vi "DriverStationSendData.vi"   [LabVIEW 2020]
doc: "This VI continously sends data from the robot to the FRC 4265 Dashboard, the joysticks, and the FIRST Driver Station. Data are only sent to the network tables when values change. Detailed sensor data are only sent when the user is currently viewing the Tune tab on the FRC 4265 Dashboard."
uses:
  586985d1-6105-46df-bd9b-6f07d21ed352.vi
  9d68b025-fd20-40c1-968a-0b15d20a54dd.vi
  423974b0-4a7b-493f-bebd-78b7d8b4919e.vi
  195aadaf-e727-4ba4-8a8c-fe9315911b93.vi
  fd66a432-e6c7-4ce8-9440-e2a32478c4e6.vi
  a01e8785-2e45-445a-ba95-97aad2eef7fd.vi
  f8967374-96a0-4ff7-9b39-d84b703c09a6.vi
  36759aca-d9c6-44a3-918a-9a0e895c718f.vi
  d2dc3f3f-39b5-4c17-a933-05bbedc8d5d9.vi
  47e8091e-0604-4560-b6ee-932fcc40f94c.vi
  040c557e-2b24-4d13-8fef-d98c711cf45f.vi
  6883bb39-9618-44d1-87fc-0a8820399f5c.vi
  c8eef334-f098-4cd9-9ea5-5d5092550f38.vi
  89115614-314f-44eb-b4c5-fafba5d31cd4.vi
  7dbbd9ae-9e42-48a3-962d-7503ed9ff88f.vi
  f31b310c-46e7-4cd5-9fe8-a6567badd324.vi
  9f98788f-6f1b-4a83-a100-7d872b9f460c.vi
  d5b4d43d-cd94-4278-ad04-5030dc28ac17.vi
  90b8ffb3-02b0-4f37-8578-c415475fcf1f.vi
  26471c2c-aca7-4047-a7cd-e40da11d04c1.vi
  839d0640-05f3-423d-909c-b7036ab13647.vi
  04c53935-f0da-44ec-a78a-2e7adf0baac3.vi
  e4b3569e-220c-43b1-9843-603dbcb8d192.vi
  0c9c2ce5-4f8f-4d2f-a61f-dde9fdddd21a.vi
  948ebb5e-1fee-45f5-b788-843df8d92f11.vi
  07cec073-88f4-4f05-94a3-d05e12405c4e.vi
  c10cd8a7-bdb7-4c92-ac5c-00af4ab7dc85.vi
  ce82ba1c-dcc2-498f-8d23-146b12230de2.vi
  6245c486-c412-4e37-a41a-fc8346b5d865.vi
  15bc976b-cae7-4018-a285-3ceb7c36b13a.vi
  cbbdf295-aa1d-4db8-8566-cac5820e4458.vi
  52d993e2-6fbc-4ee4-b085-b3f80a4c3067.vi
  5ccc8aa6-325d-4660-b060-52e30b1d582a.vi
  296afef1-bc02-48ee-92b6-09523bb21575.vi
  811948b9-57e2-4f47-a6f6-f2932d14082f.vi
  5739ca73-a30d-4c92-9c50-72d6edc45fc4.vi
  0620df73-5841-450f-a219-dd10bb38cbc0.vi
  fb087c59-fbb1-4979-ba7d-d29f083bcd8a.vi
  94826c24-d30e-4eee-b4d4-6d626a9b9fe7.vi
  fa7611ee-6daf-4341-84ec-bae2216748b8.vi
  db54ab23-5628-4d32-8d99-5ed0975ac3fe.vi
  8f6ab1f9-5983-4917-be41-7b146f8af2a0.vi
  4287b2c4-d12d-433b-80b7-0e569e2acc2b.vi
  011bd4f8-b5d7-4f12-8be3-d50395e1dcf1.vi
  f674d2d5-6a94-4f89-a0c2-325738beccea.vi
  281bad53-2b02-4799-afd8-5b44cc752506.vi
  47b7797c-6abd-448a-a8c1-ba6fc8ec09e7.vi
  65b8bab8-f184-4713-b917-96f68816fcd7.vi
  e783cd06-363b-4b9f-976c-53354950d7da.vi
  6a204843-18fb-45b9-b066-5e86b1c86445.vi
  0f67704b-983f-40f8-b984-26854eaa7ede.vi
  72a9b6b9-5c07-430f-a317-8ae0f710e1b8.vi
  d6d4123b-2723-46fe-ae0c-2abe92ccdc7f.vi
  7889d354-fa55-478c-b42d-730a5990e710.vi
  09f305fd-a7e8-43a8-8a10-94883e021016.vi
  f11304fe-b25d-4509-a679-e814399fdb49.vi
  d69f5ca2-9cc8-4f10-9e43-09bf58b41655.vi
  fa6aa2a5-b57b-4d46-802a-52895c79f189.vi
  1761f515-972c-49cd-8d46-35dcec4c579e.vi
  14433321-cc0b-4c86-996a-891af0111116.vi
  665401e1-7162-4411-af45-b6d951c7e0b0.vi
  7b6a1411-5027-49fa-871d-ec9f81e31f95.vi
  20dd8ad3-6bbc-4cac-b559-7f798e2b6680.vi
  5e95d400-1295-40c5-af46-ec5444c3a2ff.vi
  d5b53c9f-0752-48c4-83e9-94c6e20357af.vi
  a2a431f6-075f-4920-bddd-4a0a2690fbc3.vi
  755407eb-a184-43a3-8213-370691478bd6.vi
  293bca24-914b-4f92-b125-1f9f12182447.vi
  63edfc8b-2713-4fb9-bbf0-712b13f7ed91.vi
  5dc304d7-e71b-4cd2-8d9d-954937278b50.vi
  c0b3d222-824d-4eea-b194-4551ccfede72.vi
  c227876e-c49d-4561-a8c1-0ac62d9f5df0.vi
  e617f737-58a4-4889-9924-01a8da667f92.vi
  e9fd310d-87c6-4082-92c8-bcf79789ccf6.vi
  f0969710-38cf-416a-9d18-6a527ee639e4.vi
  a9076398-35a2-42a7-b542-3dd64d126b59.vi
  44842b00-b9c8-4b1f-a6e0-fc22f00ef89a.vi
  586985d1-6105-46df-bd9b-6f07d21ed352.vi/77c742ae-e671-49bb-a825-a6e8cebc9f63.vi
  9d68b025-fd20-40c1-968a-0b15d20a54dd.vi/77c742ae-e671-49bb-a825-a6e8cebc9f63.vi
  423974b0-4a7b-493f-bebd-78b7d8b4919e.vi/77c742ae-e671-49bb-a825-a6e8cebc9f63.vi
  195aadaf-e727-4ba4-8a8c-fe9315911b93.vi/77c742ae-e671-49bb-a825-a6e8cebc9f63.vi
  fd66a432-e6c7-4ce8-9440-e2a32478c4e6.vi/77c742ae-e671-49bb-a825-a6e8cebc9f63.vi
  a01e8785-2e45-445a-ba95-97aad2eef7fd.vi/77c742ae-e671-49bb-a825-a6e8cebc9f63.vi
  f8967374-96a0-4ff7-9b39-d84b703c09a6.vi/77c742ae-e671-49bb-a825-a6e8cebc9f63.vi
  36759aca-d9c6-44a3-918a-9a0e895c718f.vi/77c742ae-e671-49bb-a825-a6e8cebc9f63.vi
  d2dc3f3f-39b5-4c17-a933-05bbedc8d5d9.vi/77c742ae-e671-49bb-a825-a6e8cebc9f63.vi
  47e8091e-0604-4560-b6ee-932fcc40f94c.vi/77c742ae-e671-49bb-a825-a6e8cebc9f63.vi
  040c557e-2b24-4d13-8fef-d98c711cf45f.vi/77c742ae-e671-49bb-a825-a6e8cebc9f63.vi
  6883bb39-9618-44d1-87fc-0a8820399f5c.vi/77c742ae-e671-49bb-a825-a6e8cebc9f63.vi
  c8eef334-f098-4cd9-9ea5-5d5092550f38.vi/77c742ae-e671-49bb-a825-a6e8cebc9f63.vi
  89115614-314f-44eb-b4c5-fafba5d31cd4.vi/77c742ae-e671-49bb-a825-a6e8cebc9f63.vi
  7dbbd9ae-9e42-48a3-962d-7503ed9ff88f.vi/77c742ae-e671-49bb-a825-a6e8cebc9f63.vi
  f31b310c-46e7-4cd5-9fe8-a6567badd324.vi/77c742ae-e671-49bb-a825-a6e8cebc9f63.vi
  9f98788f-6f1b-4a83-a100-7d872b9f460c.vi/77c742ae-e671-49bb-a825-a6e8cebc9f63.vi
  d5b4d43d-cd94-4278-ad04-5030dc28ac17.vi/77c742ae-e671-49bb-a825-a6e8cebc9f63.vi
  90b8ffb3-02b0-4f37-8578-c415475fcf1f.vi/77c742ae-e671-49bb-a825-a6e8cebc9f63.vi
  26471c2c-aca7-4047-a7cd-e40da11d04c1.vi/77c742ae-e671-49bb-a825-a6e8cebc9f63.vi
  839d0640-05f3-423d-909c-b7036ab13647.vi/77c742ae-e671-49bb-a825-a6e8cebc9f63.vi
  04c53935-f0da-44ec-a78a-2e7adf0baac3.vi/77c742ae-e671-49bb-a825-a6e8cebc9f63.vi
  e4b3569e-220c-43b1-9843-603dbcb8d192.vi/77c742ae-e671-49bb-a825-a6e8cebc9f63.vi
  0c9c2ce5-4f8f-4d2f-a61f-dde9fdddd21a.vi/77c742ae-e671-49bb-a825-a6e8cebc9f63.vi
  948ebb5e-1fee-45f5-b788-843df8d92f11.vi/77c742ae-e671-49bb-a825-a6e8cebc9f63.vi
  07cec073-88f4-4f05-94a3-d05e12405c4e.vi/77c742ae-e671-49bb-a825-a6e8cebc9f63.vi
  c10cd8a7-bdb7-4c92-ac5c-00af4ab7dc85.vi/77c742ae-e671-49bb-a825-a6e8cebc9f63.vi
  ce82ba1c-dcc2-498f-8d23-146b12230de2.vi/77c742ae-e671-49bb-a825-a6e8cebc9f63.vi
  6245c486-c412-4e37-a41a-fc8346b5d865.vi/77c742ae-e671-49bb-a825-a6e8cebc9f63.vi
  15bc976b-cae7-4018-a285-3ceb7c36b13a.vi/77c742ae-e671-49bb-a825-a6e8cebc9f63.vi
  cbbdf295-aa1d-4db8-8566-cac5820e4458.vi/77c742ae-e671-49bb-a825-a6e8cebc9f63.vi
  52d993e2-6fbc-4ee4-b085-b3f80a4c3067.vi/77c742ae-e671-49bb-a825-a6e8cebc9f63.vi
  5ccc8aa6-325d-4660-b060-52e30b1d582a.vi/77c742ae-e671-49bb-a825-a6e8cebc9f63.vi
  296afef1-bc02-48ee-92b6-09523bb21575.vi/77c742ae-e671-49bb-a825-a6e8cebc9f63.vi
  811948b9-57e2-4f47-a6f6-f2932d14082f.vi/77c742ae-e671-49bb-a825-a6e8cebc9f63.vi
  5739ca73-a30d-4c92-9c50-72d6edc45fc4.vi/77c742ae-e671-49bb-a825-a6e8cebc9f63.vi
  0620df73-5841-450f-a219-dd10bb38cbc0.vi/77c742ae-e671-49bb-a825-a6e8cebc9f63.vi
  fb087c59-fbb1-4979-ba7d-d29f083bcd8a.vi/77c742ae-e671-49bb-a825-a6e8cebc9f63.vi
  94826c24-d30e-4eee-b4d4-6d626a9b9fe7.vi/77c742ae-e671-49bb-a825-a6e8cebc9f63.vi
  fa7611ee-6daf-4341-84ec-bae2216748b8.vi/77c742ae-e671-49bb-a825-a6e8cebc9f63.vi
  db54ab23-5628-4d32-8d99-5ed0975ac3fe.vi/77c742ae-e671-49bb-a825-a6e8cebc9f63.vi
  8f6ab1f9-5983-4917-be41-7b146f8af2a0.vi/77c742ae-e671-49bb-a825-a6e8cebc9f63.vi
  4287b2c4-d12d-433b-80b7-0e569e2acc2b.vi/77c742ae-e671-49bb-a825-a6e8cebc9f63.vi
  011bd4f8-b5d7-4f12-8be3-d50395e1dcf1.vi/77c742ae-e671-49bb-a825-a6e8cebc9f63.vi
  f674d2d5-6a94-4f89-a0c2-325738beccea.vi/77c742ae-e671-49bb-a825-a6e8cebc9f63.vi
  281bad53-2b02-4799-afd8-5b44cc752506.vi/77c742ae-e671-49bb-a825-a6e8cebc9f63.vi
  47b7797c-6abd-448a-a8c1-ba6fc8ec09e7.vi/77c742ae-e671-49bb-a825-a6e8cebc9f63.vi
  65b8bab8-f184-4713-b917-96f68816fcd7.vi/77c742ae-e671-49bb-a825-a6e8cebc9f63.vi
  e783cd06-363b-4b9f-976c-53354950d7da.vi/77c742ae-e671-49bb-a825-a6e8cebc9f63.vi
  6a204843-18fb-45b9-b066-5e86b1c86445.vi/77c742ae-e671-49bb-a825-a6e8cebc9f63.vi
  0f67704b-983f-40f8-b984-26854eaa7ede.vi/77c742ae-e671-49bb-a825-a6e8cebc9f63.vi
  72a9b6b9-5c07-430f-a317-8ae0f710e1b8.vi/77c742ae-e671-49bb-a825-a6e8cebc9f63.vi
  d6d4123b-2723-46fe-ae0c-2abe92ccdc7f.vi/77c742ae-e671-49bb-a825-a6e8cebc9f63.vi
  7889d354-fa55-478c-b42d-730a5990e710.vi/77c742ae-e671-49bb-a825-a6e8cebc9f63.vi
  09f305fd-a7e8-43a8-8a10-94883e021016.vi/77c742ae-e671-49bb-a825-a6e8cebc9f63.vi
  f11304fe-b25d-4509-a679-e814399fdb49.vi/77c742ae-e671-49bb-a825-a6e8cebc9f63.vi
  d69f5ca2-9cc8-4f10-9e43-09bf58b41655.vi/77c742ae-e671-49bb-a825-a6e8cebc9f63.vi
  fa6aa2a5-b57b-4d46-802a-52895c79f189.vi/77c742ae-e671-49bb-a825-a6e8cebc9f63.vi
  1761f515-972c-49cd-8d46-35dcec4c579e.vi/77c742ae-e671-49bb-a825-a6e8cebc9f63.vi
  14433321-cc0b-4c86-996a-891af0111116.vi/77c742ae-e671-49bb-a825-a6e8cebc9f63.vi
  665401e1-7162-4411-af45-b6d951c7e0b0.vi/77c742ae-e671-49bb-a825-a6e8cebc9f63.vi
  7b6a1411-5027-49fa-871d-ec9f81e31f95.vi/77c742ae-e671-49bb-a825-a6e8cebc9f63.vi
  20dd8ad3-6bbc-4cac-b559-7f798e2b6680.vi/77c742ae-e671-49bb-a825-a6e8cebc9f63.vi
  5e95d400-1295-40c5-af46-ec5444c3a2ff.vi/77c742ae-e671-49bb-a825-a6e8cebc9f63.vi
  d5b53c9f-0752-48c4-83e9-94c6e20357af.vi/77c742ae-e671-49bb-a825-a6e8cebc9f63.vi
  a2a431f6-075f-4920-bddd-4a0a2690fbc3.vi/77c742ae-e671-49bb-a825-a6e8cebc9f63.vi
  755407eb-a184-43a3-8213-370691478bd6.vi/77c742ae-e671-49bb-a825-a6e8cebc9f63.vi
  293bca24-914b-4f92-b125-1f9f12182447.vi/77c742ae-e671-49bb-a825-a6e8cebc9f63.vi
  63edfc8b-2713-4fb9-bbf0-712b13f7ed91.vi/77c742ae-e671-49bb-a825-a6e8cebc9f63.vi
  5dc304d7-e71b-4cd2-8d9d-954937278b50.vi/77c742ae-e671-49bb-a825-a6e8cebc9f63.vi
  c227876e-c49d-4561-a8c1-0ac62d9f5df0.vi/77c742ae-e671-49bb-a825-a6e8cebc9f63.vi
  e617f737-58a4-4889-9924-01a8da667f92.vi/77c742ae-e671-49bb-a825-a6e8cebc9f63.vi
  e9fd310d-87c6-4082-92c8-bcf79789ccf6.vi/77c742ae-e671-49bb-a825-a6e8cebc9f63.vi
  f0969710-38cf-416a-9d18-6a527ee639e4.vi/77c742ae-e671-49bb-a825-a6e8cebc9f63.vi
  a9076398-35a2-42a7-b542-3dd64d126b59.vi/77c742ae-e671-49bb-a825-a6e8cebc9f63.vi
  44842b00-b9c8-4b1f-a6e0-fc22f00ef89a.vi/77c742ae-e671-49bb-a825-a6e8cebc9f63.vi
  driverdata.vi
  robotconstants.vi
  <vilib>/Rock Robotics/Network Tables/NT Write String Array.vi
  <vilib>/Rock Robotics/Network Tables/NT Write String.vi
  robotprofiles.vi
  <vilib>/Rock Robotics/Network Tables/NT Write Number.vi
  robotoutputs.vi
  <vilib>/Rock Robotics/Network Tables/NT Write Boolean Array.vi
  <vilib>/Rock Robotics/Network Tables/NT Write Boolean.vi
  sensordata.vi
  <vilib>/Rock Robotics/Network Tables/NT Write Numeric Array.vi
  autonomousinfo.vi
types:
  T1 = enum16{"Robot-Oriented", "Field-Oriented", "Intake"}
  T2 = typedef "WPI_DriverStationAllianceInfo.ctl" = enum16{"Red", "Blue", "Invalid"}
  T3 = enum16{"Low Gear", "High Gear", "Transiting", "Unknown", "Force Low Gear"}
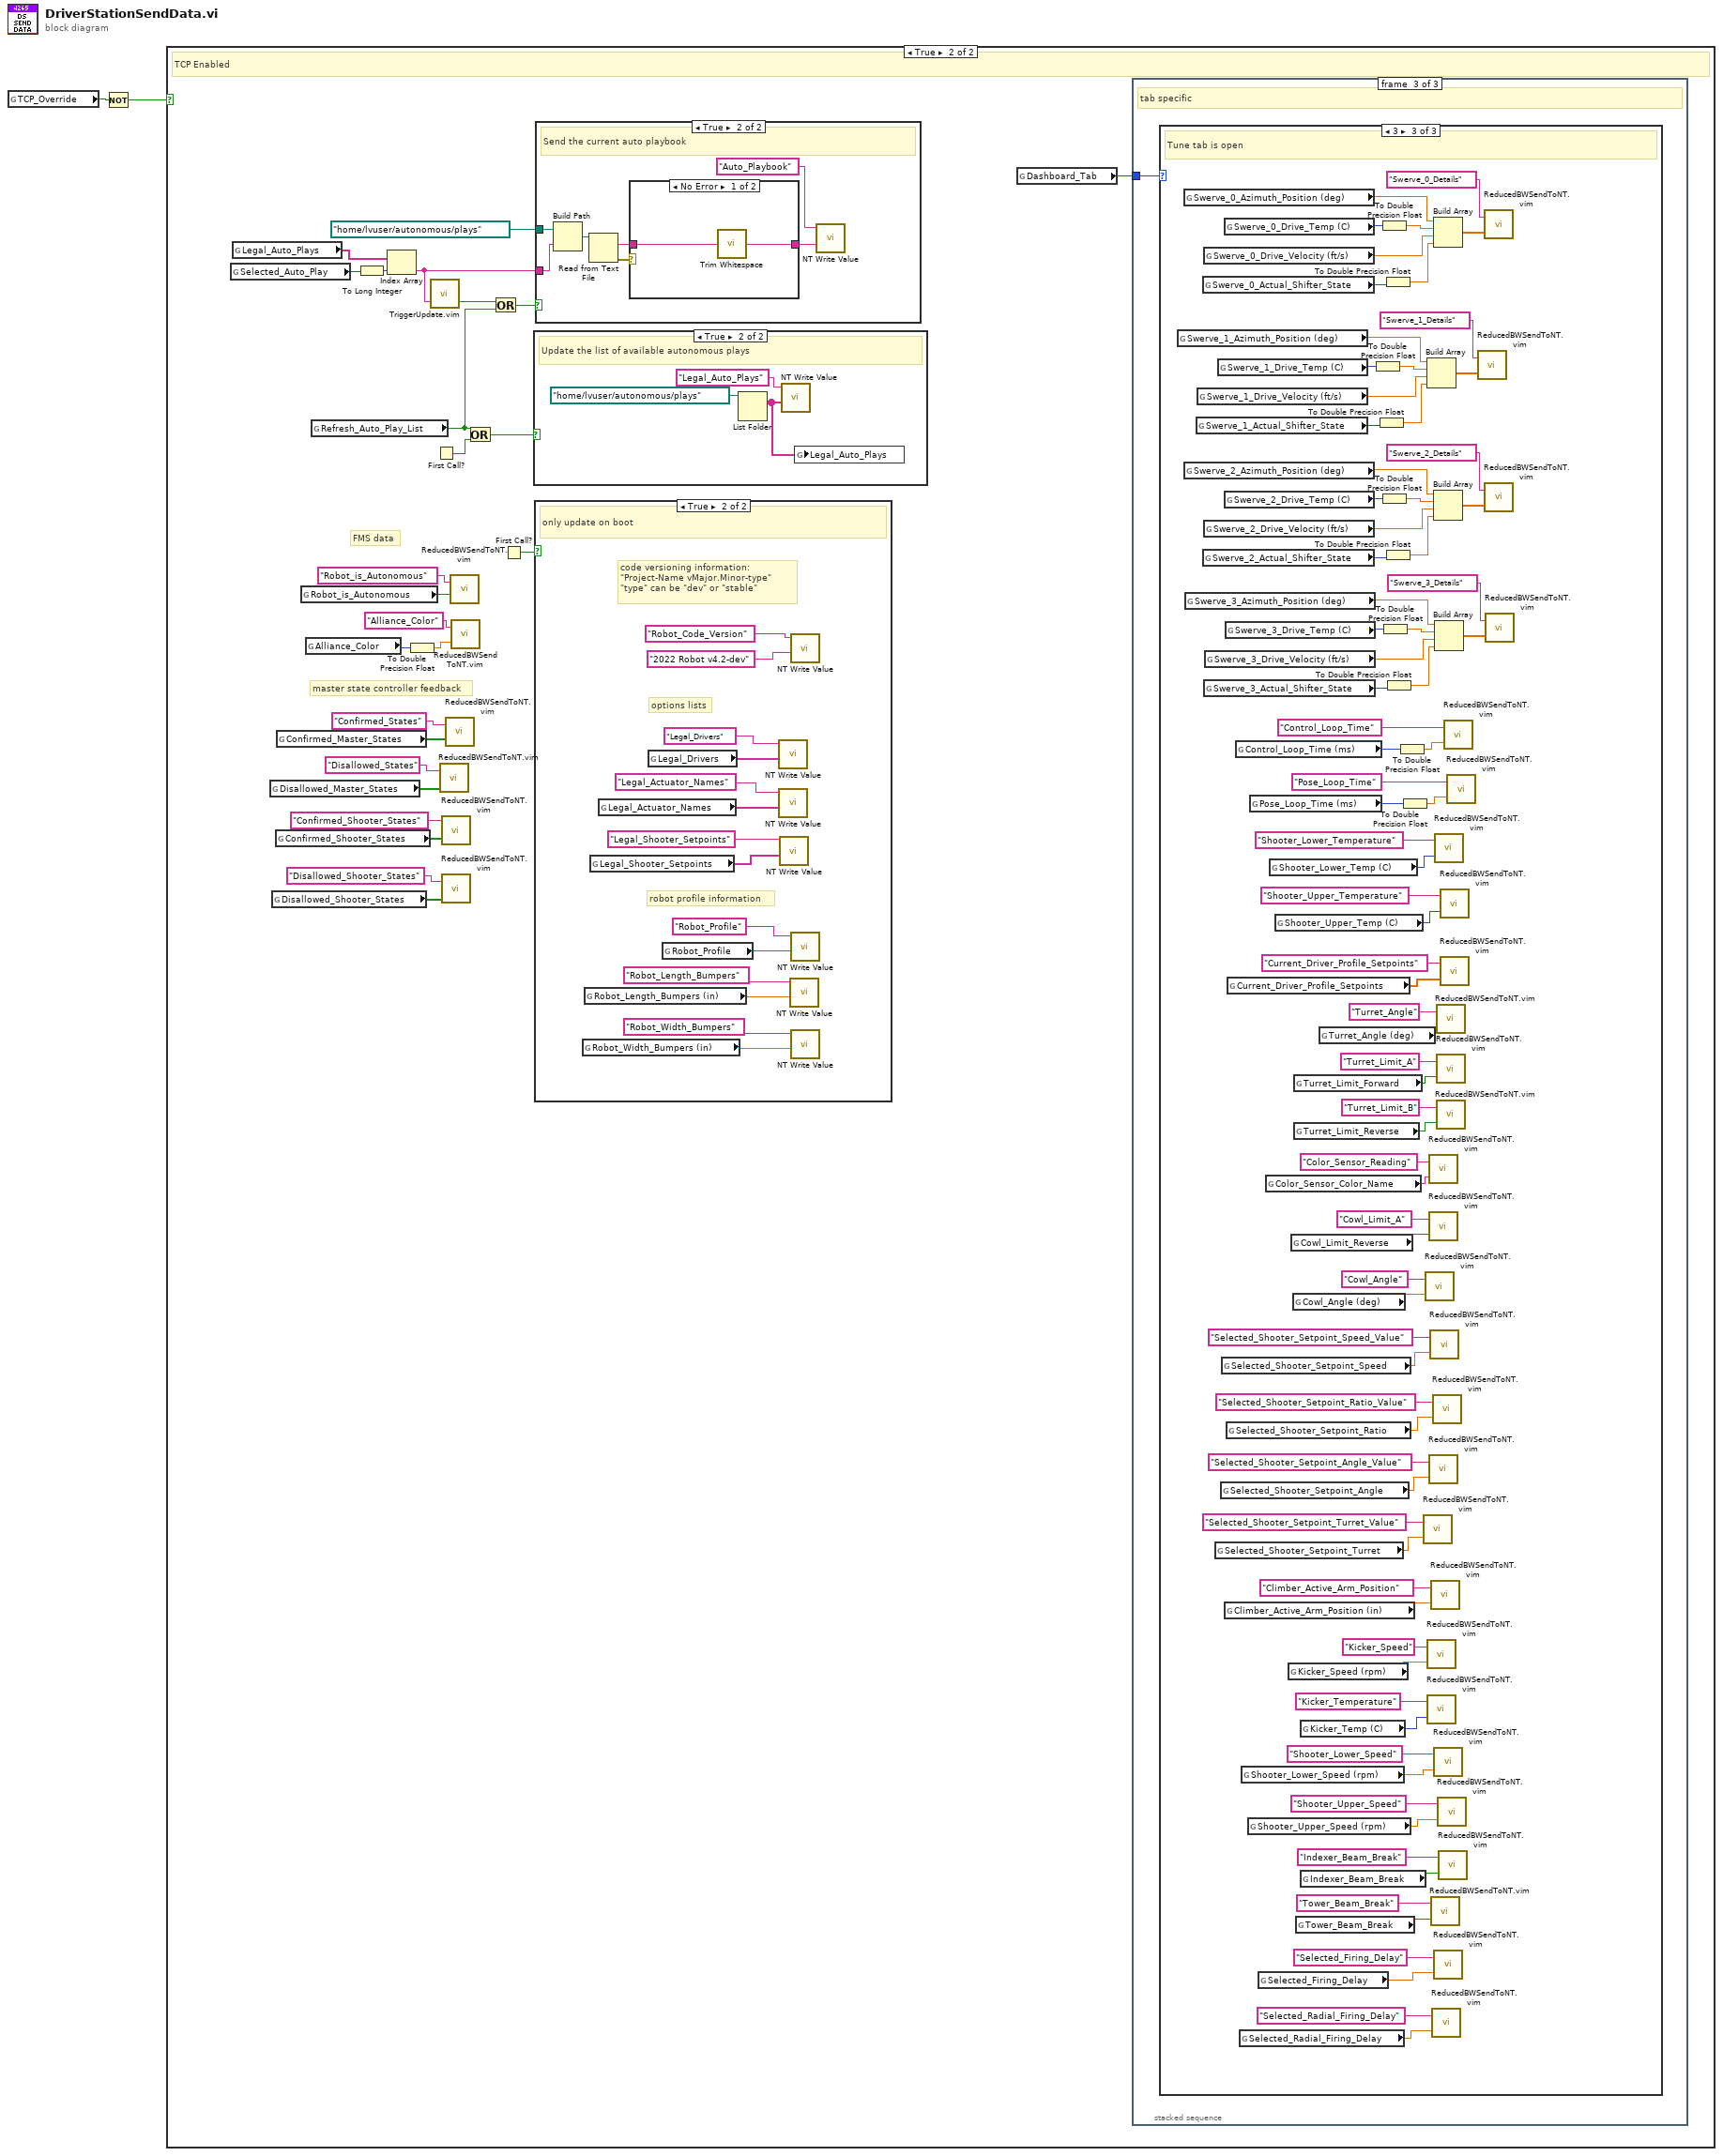
[diagram p0: block diagram]
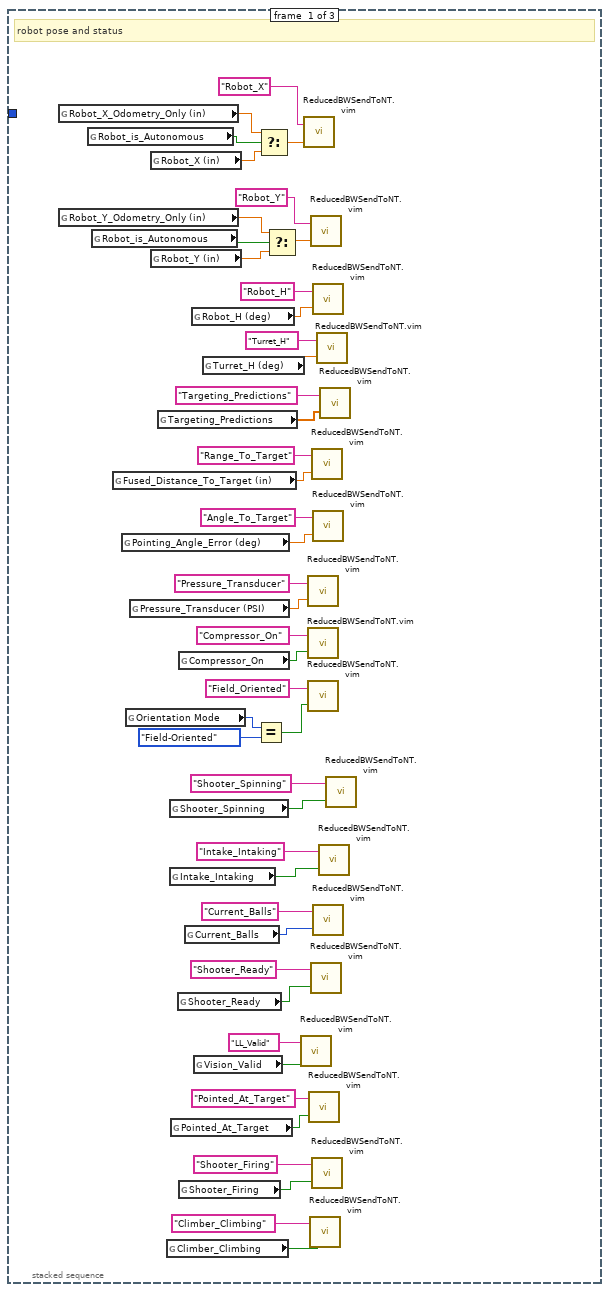
[diagram p3: hidden frame]
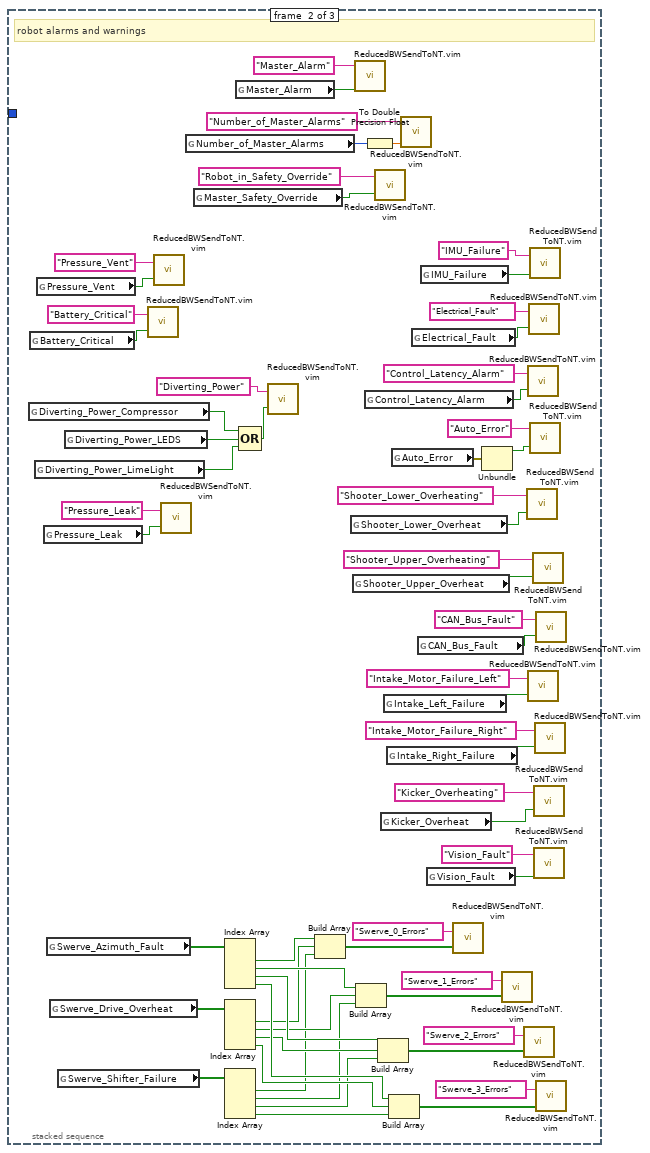
[diagram p4: hidden frame]
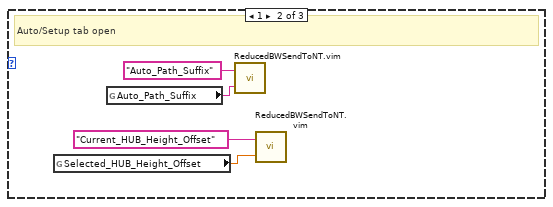
[diagram p6: hidden frame]
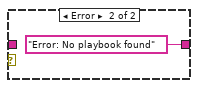
[diagram p9: hidden frame]
diagram:
  n1 = global read "driverdata.vi" "TCP_Override"() -> (w2:bool)
  n2 = Not(x=w2) -> (.not. x?=w1:bool)
  n3 = case shown="True" w1 {
    frame False {
      # "TCP Disabled"
    }
    frame True {
      # "FMS data"
      # "master state controller feedback"
      # "TCP Enabled"
      n4 = global read "driverdata.vi" "Selected_Auto_Play"() -> (w23:u16)
      n5 = global read "robotconstants.vi" "Legal_Auto_Plays"() -> (w18:string[])
      n6 = global read "robotoutputs.vi" "Disallowed_Master_States"() -> (w8:bool[])
      n7 = global read "robotoutputs.vi" "Disallowed_Shooter_States"() -> (w4:bool[])
      n8 = global read "robotoutputs.vi" "Confirmed_Shooter_States"() -> (w6:bool[])
      n9 = global read "robotoutputs.vi" "Confirmed_Master_States"() -> (w10:bool[])
      n10 = global read "driverdata.vi" "Robot_is_Autonomous"() -> (w14:bool)
      n11 = global read "driverdata.vi" "Alliance_Color"() -> (w16:T2)
      n12 = global read "driverdata.vi" "Refresh_Auto_Play_List"() -> (w19:bool)
      n13 = To Long Integer(number=w23) -> (32bit integer=w24:i32)
      n14 = Index Array(array=w18, index=w24) -> (element=w22:string)
      n15 = To Double Precision Float(number=w16) -> (double precision float=w12:dbl)
      n16 = call "TriggerUpdate.vim"("Trigger"=w22) -> ("Update"=w21:bool)  [unwired: 2 in]
      n17 = First Call?() -> (First Call?: T/F=w27:bool)
      n18 = call "ReducedBWSendToNT.vim"("Value In"=w8, "NT Name"="Disallowed_States" ("Name")) -> ()  [unwired: 1 out]
      n19 = call "ReducedBWSendToNT.vim"("Value In"=w6, "NT Name"="Confirmed_Shooter_States" ("Name")) -> ()  [unwired: 1 out]
      n20 = call "ReducedBWSendToNT.vim"("Value In"=w4, "NT Name"="Disallowed_Shooter_States" ("Name")) -> ()  [unwired: 1 out]
      n21 = call "ReducedBWSendToNT.vim"("Value In"=w10, "NT Name"="Confirmed_States" ("Name")) -> ()  [unwired: 1 out]
      n22 = call "ReducedBWSendToNT.vim"("Value In"=w14, "NT Name"="Robot_is_Autonomous") -> ()  [unwired: 1 out]
      n23 = call "ReducedBWSendToNT.vim"("Value In"=w12, "NT Name"="Alliance_Color") -> ()  [unwired: 1 out]
      n24 = Or(x=w19, y=w27) -> (x .or. y?=w26:bool)
      n25 = Or(x=w21, y=w19) -> (x .or. y?=w20:bool)
      n26 = First Call?() -> (First Call?: T/F=w17:bool)
      n27 = case shown="True" w26 {
        frame False {
        }
        frame True {
          # "Update the list of available autonomous plays"
          n28 = List Folder(path=path "/home/lvuser/autonomous/plays") -> (filenames=w247:string[])  [unwired: 3 in, 3 out]
          n29 = call-poly <vilib>:"NT Write Value.vi"("String Array"=w247, "Name"="Legal_Auto_Plays") -> ()  [unwired: 9 in, 1 out]
          n30 = global write "robotconstants.vi" "Legal_Auto_Plays"(w247) -> ()
        }
      }
      n31 = case shown="True" w17 {
        frame False {
        }
        frame True {
          # "robot profile information"
          # "options lists"
          # "code versioning information:\n\"Project-Name vMajor.Minor-type\"\n\"type\" can be \"dev\" or \"stable\""
          # "only update on boot"
          n32 = global read "robotconstants.vi" "Robot_Width_Bumpers (in)"() -> (w225:dbl)
          n33 = global read "robotconstants.vi" "Robot_Length_Bumpers (in)"() -> (w228:dbl)
          n34 = global read "robotconstants.vi" "Legal_Shooter_Setpoints"() -> (w231:string[])
          n35 = global read "robotconstants.vi" "Legal_Actuator_Names"() -> (w232:string[])
          n36 = global read "robotconstants.vi" "Legal_Drivers"() -> (w230:string[])
          n37 = global read "robotprofiles.vi" "Robot_Profile"() -> (w229:string)
          n38 = call-poly <vilib>:"NT Write Value.vi"("String Array"=w230, "Name"="Legal_Drivers") -> ()  [unwired: 9 in, 1 out]
          n39 = call-poly <vilib>:"NT Write Value.vi"("String Array"=w232, "Name"="Legal_Actuator_Names") -> ()  [unwired: 9 in, 1 out]
          n40 = call-poly <vilib>:"NT Write Value.vi"("String Array"=w231, "Name"="Legal_Shooter_Setpoints") -> ()  [unwired: 9 in, 1 out]
          n41 = call-poly <vilib>:"NT Write Value.vi"("Numeric"=w228, "Name"="Robot_Length_Bumpers") -> ()  [unwired: 9 in, 1 out]
          n42 = call-poly <vilib>:"NT Write Value.vi"("String"="2022 Robot v4.2-dev", "Name"="Robot_Code_Version") -> ()  [unwired: 9 in, 1 out]
          n43 = call-poly <vilib>:"NT Write Value.vi"("String"=w229, "Name"="Robot_Profile") -> ()  [unwired: 9 in, 1 out]
          n44 = call-poly <vilib>:"NT Write Value.vi"("Numeric"=w225, "Name"="Robot_Width_Bumpers") -> ()  [unwired: 9 in, 1 out]
        }
      }
      n45 = case shown="True" w20 {
        tunnel: path "/home/lvuser/autonomous/plays" ("path") -> [_ w243]
        tunnel: w22 -> [_ w239]
        frame False {
        }
        frame True {
          # "Send the current auto playbook"
          n46 = Build Path(base path=w243, name or relative path=w239) -> (appended path=w242:path)
          n47 = Read from Text File(file (use dialog)=w242) -> (text=w240:string, error out=w241:errorcluster)  [unwired: 3 in, 2 out]
          n48 = case shown="No Error" w241 {
            tunnel: w240 -> [w244 _]
            tunnel: [w245 "Error: No playbook found"] -> w238
            frame No Error {
              n49 = call <vilib>:"Trim Whitespace.vi"("string"=w244) -> ("trimmed string"=w245:string)  [unwired: 1 in]
            }
            frame Error {
            }
          }
          n50 = call-poly <vilib>:"NT Write Value.vi"("String"=w238, "Name"="Auto_Playbook") -> ()  [unwired: 9 in, 1 out]
        }
      }
      n51 = global read "driverdata.vi" "Dashboard_Tab"() -> (w3:i8)
      n52 = stacked-sequence {
        tunnel: w3 -> [_ _ w136]
        frame #0 {
          # "robot pose and status"
          n53 = global read "sensordata.vi" "Robot_X_Odometry_Only (in)"() -> (w66:dbl)
          n54 = global read "sensordata.vi" "Robot_Y_Odometry_Only (in)"() -> (w67:dbl)
          n55 = global read "driverdata.vi" "Robot_is_Autonomous"() -> (w70:bool)
          n56 = global read "driverdata.vi" "Robot_is_Autonomous"() -> (w71:bool)
          n57 = global read "sensordata.vi" "Fused_Distance_To_Target (in)"() -> (w59:dbl)
          n58 = global read "sensordata.vi" "Pointing_Angle_Error (deg)"() -> (w60:dbl)
          n59 = global read "robotoutputs.vi" "Orientation Mode"() -> (w50:T1)
          n60 = global read "sensordata.vi" "Pressure_Transducer (PSI)"() -> (w44:dbl)
          n61 = global read "sensordata.vi" "Robot_X (in)"() -> (w64:dbl)
          n62 = global read "sensordata.vi" "Robot_Y (in)"() -> (w65:dbl)
          n63 = global read "sensordata.vi" "Targeting_Predictions"() -> (w62:dbl[])
          n64 = global read "robotoutputs.vi" "Climber_Climbing"() -> (w33:bool)
          n65 = global read "robotoutputs.vi" "Shooter_Spinning"() -> (w46:bool)
          n66 = global read "robotoutputs.vi" "Intake_Intaking"() -> (w47:bool)
          n67 = global read "sensordata.vi" "Pointed_At_Target"() -> (w31:bool)
          n68 = global read "robotoutputs.vi" "Shooter_Ready"() -> (w49:bool)
          n69 = global read "sensordata.vi" "Compressor_On"() -> (w45:bool)
          n70 = global read "robotoutputs.vi" "Shooter_Firing"() -> (w32:bool)
          n71 = global read "sensordata.vi" "Current_Balls"() -> (w48:i16)
          n72 = global read "sensordata.vi" "Robot_H (deg)"() -> (w63:dbl)
          n73 = global read "sensordata.vi" "Vision_Valid"() -> (w43:bool)
          n74 = global read "sensordata.vi" "Turret_H (deg)"() -> (w61:dbl)
          n75 = Equal?(x=w50, y=T1."Field-Oriented") -> (x = y?=w51:bool)
          n76 = Select(t=w66, s=w70, f=w64) -> (s? t:f=w68:dbl)
          n77 = Select(t=w67, s=w71, f=w65) -> (s? t:f=w69:dbl)
          n78 = call "ReducedBWSendToNT.vim"("Value In"=w43, "NT Name"="LL_Valid" ("Name")) -> ()  [unwired: 1 out]
          n79 = call "ReducedBWSendToNT.vim"("Value In"=w68, "NT Name"="Robot_X" ("Name")) -> ()  [unwired: 1 out]
          n80 = call "ReducedBWSendToNT.vim"("Value In"=w44, "NT Name"="Pressure_Transducer" ("Name")) -> ()  [unwired: 1 out]
          n81 = call "ReducedBWSendToNT.vim"("Value In"=w45, "NT Name"="Compressor_On" ("Name")) -> ()  [unwired: 1 out]
          n82 = call "ReducedBWSendToNT.vim"("Value In"=w51, "NT Name"="Field_Oriented" ("Name")) -> ()  [unwired: 1 out]
          n83 = call "ReducedBWSendToNT.vim"("Value In"=w31, "NT Name"="Pointed_At_Target" ("Name")) -> ()  [unwired: 1 out]
          n84 = call "ReducedBWSendToNT.vim"("Value In"=w33, "NT Name"="Climber_Climbing" ("Name")) -> ()  [unwired: 1 out]
          n85 = call "ReducedBWSendToNT.vim"("Value In"=w69, "NT Name"="Robot_Y" ("Name")) -> ()  [unwired: 1 out]
          n86 = call "ReducedBWSendToNT.vim"("Value In"=w49, "NT Name"="Shooter_Ready" ("Name")) -> ()  [unwired: 1 out]
          n87 = call "ReducedBWSendToNT.vim"("Value In"=w59, "NT Name"="Range_To_Target" ("Name")) -> ()  [unwired: 1 out]
          n88 = call "ReducedBWSendToNT.vim"("Value In"=w32, "NT Name"="Shooter_Firing" ("Name")) -> ()  [unwired: 1 out]
          n89 = call "ReducedBWSendToNT.vim"("Value In"=w63, "NT Name"="Robot_H" ("Name")) -> ()  [unwired: 1 out]
          n90 = call "ReducedBWSendToNT.vim"("Value In"=w60, "NT Name"="Angle_To_Target" ("Name")) -> ()  [unwired: 1 out]
          n91 = call "ReducedBWSendToNT.vim"("Value In"=w48, "NT Name"="Current_Balls" ("Name")) -> ()  [unwired: 1 out]
          n92 = call "ReducedBWSendToNT.vim"("Value In"=w61, "NT Name"="Turret_H" ("Name")) -> ()  [unwired: 1 out]
          n93 = call "ReducedBWSendToNT.vim"("Value In"=w47, "NT Name"="Intake_Intaking" ("Name")) -> ()  [unwired: 1 out]
          n94 = call "ReducedBWSendToNT.vim"("Value In"=w62, "NT Name"="Targeting_Predictions" ("Name")) -> ()  [unwired: 1 out]
          n95 = call "ReducedBWSendToNT.vim"("Value In"=w46, "NT Name"="Shooter_Spinning" ("Name")) -> ()  [unwired: 1 out]
        }
        frame #1 {
          # "robot alarms and warnings"
          n96 = global read "robotoutputs.vi" "Diverting_Power_Compressor"() -> (w124:bool)
          n97 = global read "sensordata.vi" "Battery_Critical"() -> (w121:bool)
          n98 = global read "robotoutputs.vi" "Diverting_Power_LimeLight"() -> (w129:bool)
          n99 = global read "sensordata.vi" "Pressure_Vent"() -> (w118:bool)
          n100 = global read "sensordata.vi" "Pressure_Leak"() -> (w103:bool)
          n101 = global read "sensordata.vi" "Swerve_Azimuth_Fault"() -> (w81:bool[])
          n102 = global read "sensordata.vi" "Swerve_Drive_Overheat"() -> (w82:bool[])
          n103 = global read "sensordata.vi" "Swerve_Shifter_Failure"() -> (w83:bool[])
          n104 = global read "robotoutputs.vi" "Diverting_Power_LEDS"() -> (w125:bool)
          n105 = call "ReducedBWSendToNT.vim"("Value In"=w121, "NT Name"="Battery_Critical" ("Name")) -> ()  [unwired: 1 out]
          n106 = call "ReducedBWSendToNT.vim"("Value In"=w118, "NT Name"="Pressure_Vent" ("Name")) -> ()  [unwired: 1 out]
          n107 = call "ReducedBWSendToNT.vim"("Value In"=w103, "NT Name"="Pressure_Leak" ("Name")) -> ()  [unwired: 1 out]
          n108 = global read "robotoutputs.vi" "Number_of_Master_Alarms"() -> (w134:i32)
          n109 = global read "driverdata.vi" "Master_Safety_Override"() -> (w130:bool)
          n110 = Index Array(array=w81) -> (element #1=w84:bool, element #2=w87:bool, element #3=w90:bool, element #4=w93:bool)  [unwired: 4 in]
          n111 = Index Array(array=w82) -> (element #1=w85:bool, element #2=w88:bool, element #3=w91:bool, element #4=w94:bool)  [unwired: 4 in]
          n112 = Index Array(array=w83) -> (element #1=w86:bool, element #2=w89:bool, element #3=w92:bool, element #4=w95:bool)  [unwired: 4 in]
          n113 = global read "robotoutputs.vi" "Master_Alarm"() -> (w133:bool)
          n114 = Compound Arithmetic op=OR(w124, w125, w129) -> (w123:bool)
          n115 = call "ReducedBWSendToNT.vim"("Value In"=w123, "NT Name"="Diverting_Power" ("Name")) -> ()  [unwired: 1 out]
          n116 = Build Array(w84, w85, w86) -> (w96:bool[])
          n117 = global read "sensordata.vi" "Shooter_Lower_Overheat"() -> (w127:bool)
          n118 = global read "sensordata.vi" "Shooter_Upper_Overheat"() -> (w128:bool)
          n119 = call "ReducedBWSendToNT.vim"("Value In"=w133, "NT Name"="Master_Alarm" ("Name")) -> ()  [unwired: 1 out]
          n120 = Build Array(w87, w88, w89) -> (w97:bool[])
          n121 = To Double Precision Float(number=w134) -> (double precision float=w135:dbl)
          n122 = global read "sensordata.vi" "Control_Latency_Alarm"() -> (w122:bool)
          n123 = call "ReducedBWSendToNT.vim"("Value In"=w130, "NT Name"="Robot_in_Safety_Override" ("Name")) -> ()  [unwired: 1 out]
          n124 = Build Array(w90, w91, w92) -> (w98:bool[])
          n125 = global read "sensordata.vi" "Kicker_Overheat"() -> (w102:bool)
          n126 = global read "sensordata.vi" "Intake_Left_Failure"() -> (w100:bool)
          n127 = global read "sensordata.vi" "Intake_Right_Failure"() -> (w101:bool)
          n128 = Build Array(w93, w94, w95) -> (w99:bool[])
          n129 = global read "autonomousinfo.vi" "Auto_Error"() -> (w116:errorcluster)
          n130 = call "ReducedBWSendToNT.vim"("Value In"=w135, "NT Name"="Number_of_Master_Alarms" ("Name")) -> ()  [unwired: 1 out]
          n131 = global read "sensordata.vi" "Electrical_Fault"() -> (w120:bool)
          n132 = global read "sensordata.vi" "CAN_Bus_Fault"() -> (w126:bool)
          n133 = global read "sensordata.vi" "IMU_Failure"() -> (w119:bool)
          n134 = global read "sensordata.vi" "Vision_Fault"() -> (w104:bool)
          n135 = call "ReducedBWSendToNT.vim"("Value In"=w96, "NT Name"="Swerve_0_Errors") -> ()  [unwired: 1 out]
          n136 = Unbundle(w116) -> ("status"=w117:bool)  [unwired: 2 out]
          n137 = call "ReducedBWSendToNT.vim"("Value In"=w97, "NT Name"="Swerve_1_Errors") -> ()  [unwired: 1 out]
          n138 = call "ReducedBWSendToNT.vim"("Value In"=w98, "NT Name"="Swerve_2_Errors") -> ()  [unwired: 1 out]
          n139 = call "ReducedBWSendToNT.vim"("Value In"=w127, "NT Name"="Shooter_Lower_Overheating" ("Name")) -> ()  [unwired: 1 out]
          n140 = call "ReducedBWSendToNT.vim"("Value In"=w122, "NT Name"="Control_Latency_Alarm" ("Name")) -> ()  [unwired: 1 out]
          n141 = call "ReducedBWSendToNT.vim"("Value In"=w100, "NT Name"="Intake_Motor_Failure_Left" ("Name")) -> ()  [unwired: 1 out]
          n142 = call "ReducedBWSendToNT.vim"("Value In"=w120, "NT Name"="Electrical_Fault" ("Name")) -> ()  [unwired: 1 out]
          n143 = call "ReducedBWSendToNT.vim"("Value In"=w119, "NT Name"="IMU_Failure" ("Name")) -> ()  [unwired: 1 out]
          n144 = call "ReducedBWSendToNT.vim"("Value In"=w117, "NT Name"="Auto_Error" ("Name")) -> ()  [unwired: 1 out]
          n145 = call "ReducedBWSendToNT.vim"("Value In"=w128, "NT Name"="Shooter_Upper_Overheating" ("Name")) -> ()  [unwired: 1 out]
          n146 = call "ReducedBWSendToNT.vim"("Value In"=w102, "NT Name"="Kicker_Overheating" ("Name")) -> ()  [unwired: 1 out]
          n147 = call "ReducedBWSendToNT.vim"("Value In"=w104, "NT Name"="Vision_Fault" ("Name")) -> ()  [unwired: 1 out]
          n148 = call "ReducedBWSendToNT.vim"("Value In"=w101, "NT Name"="Intake_Motor_Failure_Right" ("Name")) -> ()  [unwired: 1 out]
          n149 = call "ReducedBWSendToNT.vim"("Value In"=w126, "NT Name"="CAN_Bus_Fault" ("Name")) -> ()  [unwired: 1 out]
          n150 = call "ReducedBWSendToNT.vim"("Value In"=w99, "NT Name"="Swerve_3_Errors") -> ()  [unwired: 1 out]
        }
        frame #2 {
          # "tab specific"
          n151 = case shown="3" w136 {
            frame 0, Default {
              # "no tab open"
            }
            frame 1 {
              # "Auto/Setup tab open"
              n152 = global read "robotoutputs.vi" "Selected_HUB_Height_Offset"() -> (w138:dbl)
              n153 = global read "autonomousinfo.vi" "Auto_Path_Suffix"() -> (w140:string)
              n154 = call "ReducedBWSendToNT.vim"("Value In"=w140, "NT Name"="Auto_Path_Suffix" ("Name")) -> ()  [unwired: 1 out]
              n155 = call "ReducedBWSendToNT.vim"("Value In"=w138, "NT Name"="Current_HUB_Height_Offset" ("Name")) -> ()  [unwired: 1 out]
            }
            frame 3 {
              # "Tune tab is open"
              n156 = global read "sensordata.vi" "Swerve_1_Azimuth_Position (deg)"() -> (w202:dbl)
              n157 = global read "sensordata.vi" "Swerve_0_Azimuth_Position (deg)"() -> (w210:dbl)
              n158 = global read "sensordata.vi" "Swerve_2_Azimuth_Position (deg)"() -> (w194:dbl)
              n159 = global read "sensordata.vi" "Swerve_3_Azimuth_Position (deg)"() -> (w186:dbl)
              n160 = global read "sensordata.vi" "Swerve_1_Actual_Shifter_State"() -> (w198:T3)
              n161 = global read "sensordata.vi" "Swerve_1_Drive_Velocity (ft/s)"() -> (w201:dbl)
              n162 = global read "sensordata.vi" "Swerve_0_Actual_Shifter_State"() -> (w206:T3)
              n163 = global read "sensordata.vi" "Swerve_2_Actual_Shifter_State"() -> (w190:T3)
              n164 = global read "sensordata.vi" "Swerve_0_Drive_Velocity (ft/s)"() -> (w209:dbl)
              n165 = global read "sensordata.vi" "Swerve_2_Drive_Velocity (ft/s)"() -> (w193:dbl)
              n166 = global read "sensordata.vi" "Swerve_3_Actual_Shifter_State"() -> (w182:T3)
              n167 = global read "sensordata.vi" "Swerve_3_Drive_Velocity (ft/s)"() -> (w185:dbl)
              n168 = global read "robotoutputs.vi" "Selected_Shooter_Setpoint_Turret"() -> (w143:dbl)
              n169 = global read "sensordata.vi" "Swerve_1_Drive_Temp (C)"() -> (w200:u8)
              n170 = global read "robotoutputs.vi" "Selected_Shooter_Setpoint_Angle"() -> (w161:dbl)
              n171 = global read "robotoutputs.vi" "Selected_Shooter_Setpoint_Speed"() -> (w165:dbl)
              n172 = global read "sensordata.vi" "Swerve_0_Drive_Temp (C)"() -> (w208:u8)
              n173 = global read "sensordata.vi" "Swerve_2_Drive_Temp (C)"() -> (w192:u8)
              n174 = global read "sensordata.vi" "Climber_Active_Arm_Position (in)"() -> (w159:dbl)
              n175 = global read "sensordata.vi" "Swerve_3_Drive_Temp (C)"() -> (w184:u8)
              n176 = global read "robotoutputs.vi" "Selected_Shooter_Setpoint_Ratio"() -> (w163:dbl)
              n177 = global read "robotoutputs.vi" "Current_Driver_Profile_Setpoints"() -> (w212:dbl[])
              n178 = global read "sensordata.vi" "Control_Loop_Time (ms)"() -> (w222:u32)
              n179 = global read "robotoutputs.vi" "Selected_Radial_Firing_Delay"() -> (w142:dbl)
              n180 = global read "sensordata.vi" "Shooter_Lower_Speed (rpm)"() -> (w154:dbl)
              n181 = global read "sensordata.vi" "Shooter_Upper_Speed (rpm)"() -> (w151:dbl)
              n182 = global read "sensordata.vi" "Pose_Loop_Time (ms)"() -> (w219:u32)
              n183 = global read "robotoutputs.vi" "Selected_Firing_Delay"() -> (w146:dbl)
              n184 = global read "sensordata.vi" "Color_Sensor_Color_Name"() -> (w172:string)
              n185 = global read "sensordata.vi" "Shooter_Lower_Temp (C)"() -> (w216:u8)
              n186 = global read "sensordata.vi" "Shooter_Upper_Temp (C)"() -> (w214:u8)
              n187 = global read "sensordata.vi" "Kicker_Speed (rpm)"() -> (w157:dbl)
              n188 = global read "sensordata.vi" "Cowl_Limit_Reverse"() -> (w169:bool)
              n189 = global read "sensordata.vi" "Cowl_Angle (deg)"() -> (w168:dbl)
              n190 = global read "sensordata.vi" "Turret_Limit_Forward"() -> (w176:bool)
              n191 = global read "sensordata.vi" "Turret_Limit_Reverse"() -> (w174:bool)
              n192 = global read "sensordata.vi" "Tower_Beam_Break"() -> (w150:bool)
              n193 = global read "sensordata.vi" "Kicker_Temp (C)"() -> (w156:u8)
              n194 = global read "sensordata.vi" "Indexer_Beam_Break"() -> (w149:bool)
              n195 = global read "sensordata.vi" "Turret_Angle (deg)"() -> (w178:dbl)
              n196 = To Double Precision Float(number=w200) -> (double precision float=w199:dbl)
              n197 = To Double Precision Float(number=w198) -> (double precision float=w197:dbl)
              n198 = To Double Precision Float(number=w208) -> (double precision float=w207:dbl)
              n199 = To Double Precision Float(number=w192) -> (double precision float=w191:dbl)
              n200 = To Double Precision Float(number=w184) -> (double precision float=w183:dbl)
              n201 = To Double Precision Float(number=w206) -> (double precision float=w205:dbl)
              n202 = To Double Precision Float(number=w190) -> (double precision float=w189:dbl)
              n203 = To Double Precision Float(number=w182) -> (double precision float=w181:dbl)
              n204 = To Double Precision Float(number=w222) -> (double precision float=w220:dbl)
              n205 = To Double Precision Float(number=w219) -> (double precision float=w217:dbl)
              n206 = call "ReducedBWSendToNT.vim"("Value In"=w143, "NT Name"="Selected_Shooter_Setpoint_Turret_Value" ("Name")) -> ()  [unwired: 1 out]
              n207 = call "ReducedBWSendToNT.vim"("Value In"=w168, "NT Name"="Cowl_Angle" ("Name")) -> ()  [unwired: 1 out]
              n208 = Build Array(w202, w199, w201, w197) -> (w196:dbl[])
              n209 = call "ReducedBWSendToNT.vim"("Value In"=w157, "NT Name"="Kicker_Speed" ("Name")) -> ()  [unwired: 1 out]
              n210 = call "ReducedBWSendToNT.vim"("Value In"=w156, "NT Name"="Kicker_Temperature" ("Name")) -> ()  [unwired: 1 out]
              n211 = call "ReducedBWSendToNT.vim"("Value In"=w172, "NT Name"="Color_Sensor_Reading" ("Name")) -> ()  [unwired: 1 out]
              n212 = call "ReducedBWSendToNT.vim"("Value In"=w169, "NT Name"="Cowl_Limit_A" ("Name")) -> ()  [unwired: 1 out]
              n213 = call "ReducedBWSendToNT.vim"("Value In"=w161, "NT Name"="Selected_Shooter_Setpoint_Angle_Value" ("Name")) -> ()  [unwired: 1 out]
              n214 = call "ReducedBWSendToNT.vim"("Value In"=w165, "NT Name"="Selected_Shooter_Setpoint_Speed_Value" ("Name")) -> ()  [unwired: 1 out]
              n215 = call "ReducedBWSendToNT.vim"("Value In"=w159, "NT Name"="Climber_Active_Arm_Position" ("Name")) -> ()  [unwired: 1 out]
              n216 = call "ReducedBWSendToNT.vim"("Value In"=w150, "NT Name"="Tower_Beam_Break" ("Name")) -> ()  [unwired: 1 out]
              n217 = call "ReducedBWSendToNT.vim"("Value In"=w142, "NT Name"="Selected_Radial_Firing_Delay" ("Name")) -> ()  [unwired: 1 out]
              n218 = call "ReducedBWSendToNT.vim"("Value In"=w163, "NT Name"="Selected_Shooter_Setpoint_Ratio_Value" ("Name")) -> ()  [unwired: 1 out]
              n219 = Build Array(w210, w207, w209, w205) -> (w204:dbl[])
              n220 = Build Array(w194, w191, w193, w189) -> (w188:dbl[])
              n221 = call "ReducedBWSendToNT.vim"("Value In"=w154, "NT Name"="Shooter_Lower_Speed" ("Name")) -> ()  [unwired: 1 out]
              n222 = call "ReducedBWSendToNT.vim"("Value In"=w146, "NT Name"="Selected_Firing_Delay" ("Name")) -> ()  [unwired: 1 out]
              n223 = Build Array(w186, w183, w185, w181) -> (w180:dbl[])
              n224 = call "ReducedBWSendToNT.vim"("Value In"=w216, "NT Name"="Shooter_Lower_Temperature" ("Name")) -> ()  [unwired: 1 out]
              n225 = call "ReducedBWSendToNT.vim"("Value In"=w178, "NT Name"="Turret_Angle" ("Name")) -> ()  [unwired: 1 out]
              n226 = call "ReducedBWSendToNT.vim"("Value In"=w176, "NT Name"="Turret_Limit_A" ("Name")) -> ()  [unwired: 1 out]
              n227 = call "ReducedBWSendToNT.vim"("Value In"=w174, "NT Name"="Turret_Limit_B" ("Name")) -> ()  [unwired: 1 out]
              n228 = call "ReducedBWSendToNT.vim"("Value In"=w151, "NT Name"="Shooter_Upper_Speed" ("Name")) -> ()  [unwired: 1 out]
              n229 = call "ReducedBWSendToNT.vim"("Value In"=w149, "NT Name"="Indexer_Beam_Break" ("Name")) -> ()  [unwired: 1 out]
              n230 = call "ReducedBWSendToNT.vim"("Value In"=w214, "NT Name"="Shooter_Upper_Temperature" ("Name")) -> ()  [unwired: 1 out]
              n231 = call "ReducedBWSendToNT.vim"("Value In"=w212, "NT Name"="Current_Driver_Profile_Setpoints" ("Name")) -> ()  [unwired: 1 out]
              n232 = call "ReducedBWSendToNT.vim"("Value In"=w220, "NT Name"="Control_Loop_Time" ("Name")) -> ()  [unwired: 1 out]
              n233 = call "ReducedBWSendToNT.vim"("Value In"=w217, "NT Name"="Pose_Loop_Time" ("Name")) -> ()  [unwired: 1 out]
              n234 = call "ReducedBWSendToNT.vim"("Value In"=w196, "NT Name"="Swerve_1_Details") -> ()  [unwired: 1 out]
              n235 = call "ReducedBWSendToNT.vim"("Value In"=w204, "NT Name"="Swerve_0_Details") -> ()  [unwired: 1 out]
              n236 = call "ReducedBWSendToNT.vim"("Value In"=w188, "NT Name"="Swerve_2_Details") -> ()  [unwired: 1 out]
              n237 = call "ReducedBWSendToNT.vim"("Value In"=w180, "NT Name"="Swerve_3_Details") -> ()  [unwired: 1 out]
            }
          }
        }
      }
    }
  }
